vi "IT8800-Configure Protection.vi"(5 "Enable UVP":bool, 7 "Enable Trip":bool, 8 "error in":errorcluster, 9 "Protection Limit (0)":dbl, 10 "Protection Type (0:OCP)":u16(ring) items=["Over Current Protection (OCP)", "Over Power Protection (OPP)", "Under Voltage Protection (UVP)"], 11 "IT8800 Setting In In":T1={"VISA Resource Name"="", "Baud Rate"=19200, "Stop Bits"=20, "Wait For Read(ms)"=0, "Interface Type"=enum."GPIB", "Limits"=[]} {"Stop Bits" items=["1.0"=10, "2.0"=20]; "Baud Rate" items=["2400"=2400, "4800"=4800, "9600"=9600, "19200"=19200]}) -> (0 "error out":errorcluster, 3 "IT8800 Setting In Out":T1={"VISA Resource Name"="", "Baud Rate"=19200, "Stop Bits"=20, "Wait For Read(ms)"=0, "Interface Type"=enum."GPIB", "Limits"=[]} {"Stop Bits" items=["1.0"=10, "2.0"=20]; "Baud Rate" items=["2400"=2400, "4800"=4800, "9600"=9600, "19200"=19200]})   [LabVIEW 2018]
doc: "Configures current, power or voltage protection. Whenever the current, power or voltage reaches the limit specified, it will either limit or turn off the load."
uses:
  Data Def/IT8800-Setting.ctl
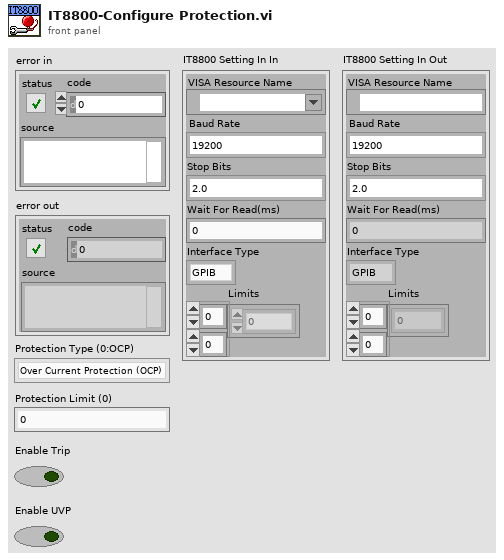
[diagram p1: front panel]
types:
  T1 = typedef "IT8800-Setting.ctl" = cluster{"VISA Resource Name":refnum<visa-resource-name>, "Baud Rate":u32, "Stop Bits":u16, "Wait For Read(ms)":u32, "Interface Type":enum16{"Unknow", "GPIB", "VXI", "GPIB-VXI", "Serial", "PXI", "TCPIP", "USB", "FireWire"}, "Limits":dbl[][]}
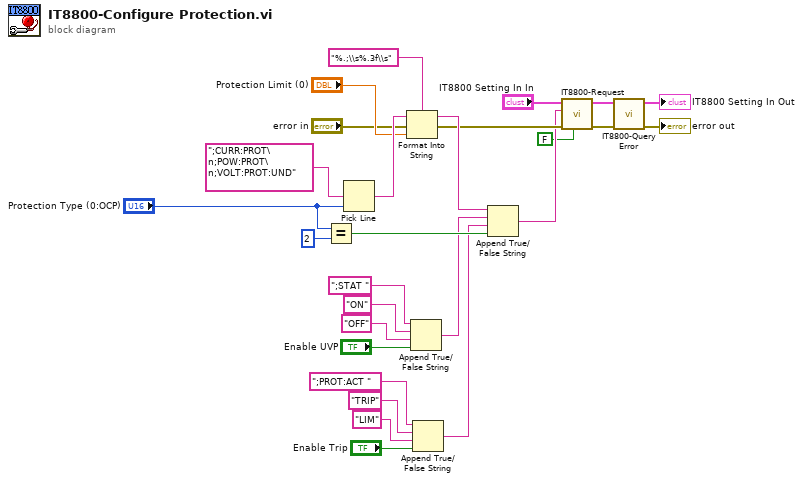
[diagram p0: block diagram]
diagram:
  n1 = Equal?(x="Protection Type (0:OCP)", y=u16 2) -> (x = y?=w19:bool)
  n2 = Pick Line(multi-line string=";CURR:PROT\n;POW:PROT\n;VOLT:PROT:UND", line index="Protection Type (0:OCP)") -> (output string=w25:string)  [unwired: 1 in]
  n3 = Format Into String(format string="%.;\\s%.3f\\s", initial string=w25, error in="error in", "Protection Limit (0)") -> (resulting string=w15:string, error out=w5:errorcluster)
  n4 = Append True/False String(1:"Enable UVP", 2:"OFF" ("false string"), 3:"ON" ("true string"), 4:";STAT " ("string (\"\")")) -> (0:w17:string)
  n5 = Append True/False String(1:"Enable Trip", 2:"LIM" ("false string"), 3:"TRIP" ("true string"), 4:";PROT:ACT " ("false string")) -> (0:w16:string)
  n6 = Append True/False String(1:w19, 2:w16, 3:w17, 4:w15) -> (0:w4:string)
  n7 = call "IT8800-Request.vi"("Response?"=FALSE, "error in"=w5, "Command"=w4, "IT8800 Setting In In"="IT8800 Setting In In") -> ("error out"=w7:errorcluster, "IT8800 Setting In Out"=w6:T1)  [unwired: 5 in, 1 out]
  n8 = call "IT8800-Query Error.vi"("error in"=w7, "IT8800 Setting In In"=w6) -> ("error out"=→"error out":errorcluster, "IT8800 Setting In Out"=→"IT8800 Setting In Out":T1)  [unwired: 8 in]
